vi "Generate_Pos_Const.vi"(8 "error in (no error)":errorcluster, 9 "location":T1, 11 "VI in":refnum<vi>) -> (0 "error out":errorcluster, 2 "Terminal":refnum<vi>, 3 "New Object Reference":refnum<vi>)   [LabVIEW 2025]
uses:
  <vilib>/Utility/miscctls.llb/LVPointTypeDef.ctl
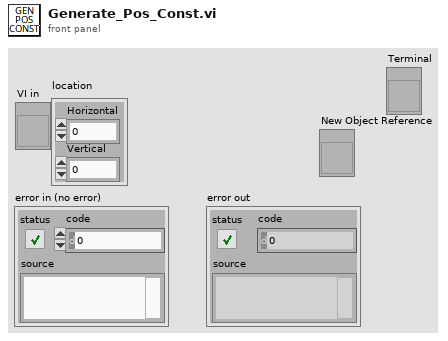
[diagram p1: front panel]
types:
  T1 = typedef "LVPointTypeDef.ctl" = cluster{"Horizontal":i16, "Vertical":i16}
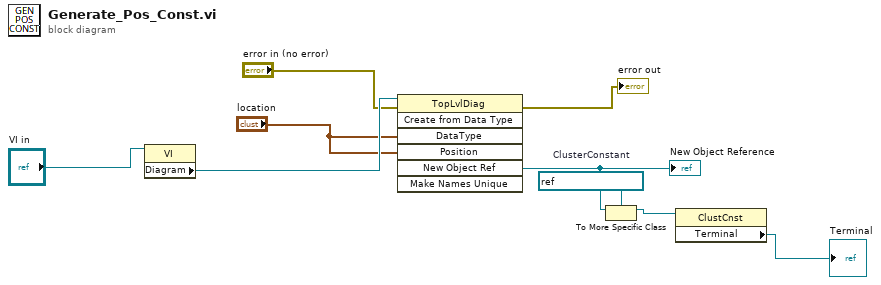
[diagram p0: block diagram]
diagram:
  w3 = refnum<vi> refnum  # ClusterConstant
  n1 = property class="VI"(reference="VI in") -> ("Diagram"=w9:refnum<vi>)  [unwired: 1 in, 2 out]
  n2 = invoke class="TopLvlDiag" method="Create from Data Type"(reference=w9, error in="error in (no error)", "DataType"="location", "Position"="location") -> (error out=→"error out":errorcluster, "New Object Ref"=w4:refnum<vi>)  [unwired: 3 in, 5 out]
  "New Object Reference" <- w4
  n3 = To More Specific Class(target class=w3, reference=w4) -> (specific class reference=w2:refnum<vi>)  [unwired: 1 in, 1 out]
  n4 = property class="ClustCnst"(reference=w2) -> ("Terminal"=→"Terminal":refnum<vi>)  [unwired: 1 in, 2 out]
